vi "Shutdown.vi"(8 "error in (no error)":errorcluster, 11 "Plugin in":refnum<class "Plugin.lvclass">) -> (0 "error out":errorcluster, 3 "Plugin out":refnum<class "Plugin.lvclass">)   [LabVIEW 2019, in "DSF Core.lvlib" / "Plugin.lvclass"]
uses:
  Plugin.lvclass
  Plugin.lvclass/Plugin.ctl
  Interface/Interface.lvclass/Interface.ctl
  Interface/Errors.vi
  Interface/Dispatcher/Invalid Response.vi
  Interface/Plugin/Class Name.vi
  Interface/Plugin/Wait For.vi
  Interface/Plugin/Wait For Plugin Response.vi
  Interface/Plugin/Send.vi
  Interface/Plugin/Send Plugin Command.vi
  <vilib>/NI/Memory Manager/VIs/Write String to Source.vi
  Interface/New Interface Error.vi
  Interface/Wait For Response.vi
  Interface/Dispatcher/Response Timeout.vi
  Interface/Send Command.vi
  Interface/Dispatcher/Command Timeout.vi
  <vilib>/NI/Memory Manager/VIs/New Error Cluster.vi
  <vilib>/NI/Memory Manager/VIs/New Error Cluster (512B).vi
  <vilib>/NI/Memory Manager/VIs/Set Error Code.vi
  <vilib>/NI/Memory Manager/VIs/Set Error Status.vi
  <vilib>/NI/Memory Manager/VIs/Set Error Source.vi
  Interface/Interface Error Info.vi
  Interface/Read RT FIFO.vi
  Interface/Write RT FIFO.vi
  VIs/Constants/Constants.vi
  VIs/Constants/Base Error Code.vi
  Interface/Interface Error Offset.vi
  Interface/Plugin/Plugin Interface.lvclass
  C:/Dev/GitHub/niveristand-data-sharing-framework-custom-device/Core/Classes/Interface/Interface.lvclass
  VIs/VI Name.vi
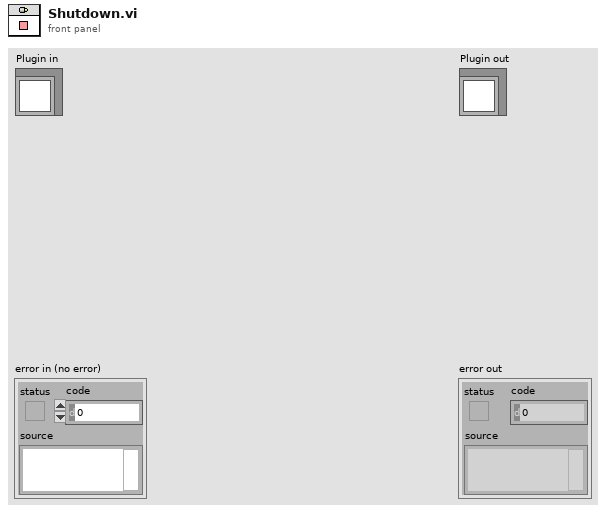
[diagram p1: front panel]
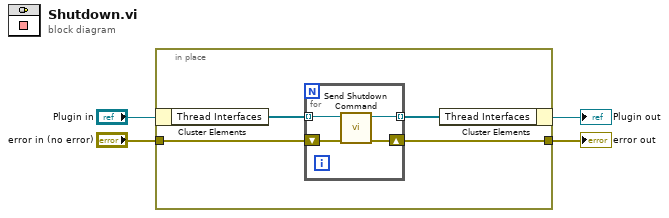
[diagram p0: block diagram]
diagram:
  n1 = in-place {
    in-place-border: "error in (no error)" -> [w8]
    in-place-border: [w7] -> w1
    n2 = in-place-cluster #1("Plugin in") -> ("Thread Interfaces"=w6:refnum<class "Plugin Interface.lvclass">[])
    n3 = for {
      shift-right: [w9] -> w7
      shift-left: w8 -> [w10]
      tunnel: [w11] -> w5 mode=indexing
      tunnel: w6 -> [w12] mode=indexing
      n4 = call "Send Shutdown Command.vi"("error in (no error)"=w10, "Plugin Interface in"=w12) -> ("error out"=w9:errorcluster, "Plugin Interface out"=w11:refnum<class "Plugin Interface.lvclass">)  [unwired: 8 in]
    }
    n5 = in-place-cluster #1("Thread Interfaces"=w5) -> (→"Plugin out":refnum<class "Plugin.lvclass">)
  }
  "error out" <- w1
